vi "Curtin1.vi"() -> ()   [LabVIEW 2022 SP3]
uses:
  ViolinSubs/Curtin1_Label.ctl
  ViolinSubs/GraphType.ctl
  <vilib>/Utility/miscctls.llb/LVPoint32TypeDef.ctl
  ViolinSubs/Mic/Mic_Global.vi
  ViolinSubs/Perspective/subs/Perspective_Globals.vi
  <vilib>/Platform/browser.llb/Open URL in Default Browser (string).vi
panel:
  in  "microphone":bool
  in  "Device":u16(ring) items=["BuerginBase Microphone", "MacBook Pro Microphone", "Reincubate", "Microsoft Teams Audio", "Jump Desktop Microphone", "Jump Desktop Audio", "ZoomAudioDevice"]
  out "comma?":bool
  out "startX":i32
  out "Ctrl":bool
  out "beta":string
  in  "Settings":u16(ring) items=["Settings...", "Preferences", "Templates", "Calibrations", "Live View", "Motor Cntrl"]
  in  "ScratchPads":u16(ring) items=["Scratch...", "Admittance Scratchpad", "Radiation ScratchPad", "ScratchPad", "TapTones ScratchPad"]
  in  "New Test":u16(ring) items=["New Test...", "Admittance H", "JC H 12 radiation", "JC H 7 radiation", "JC HV 24 radiation"]
  in  "Help":bool
  in  "About":bool
  in  "Start":bool
  in  "email":bool
  in  "Interpret":bool
  in  "Force YRescale":bool
  out "Complex Out":cluster{dbl, "df":dbl, cdb[]}[](array[cluster])
  out "# selected":i32
  in  "Fun":bool
  out "Version":string
  in  "Preferences":bool
  in  "Set Colors":bool
  in  "Colors":u16(ring) items=["Name Current...", "Last Saved", "24 Colors"]
  in  "Share":bool
  in  "Undo":bool
  in  "Clear All":bool
  in  "select all":bool
  in  "deselect":bool
  in  "Clear":bool
  in  "Lists":bool
  in  "Browse":bool
  in  "Search":bool
  in  "Redo":bool
  in  "Files":T1[](array[typedef])
  in  "zoom":bool
  in  "Mouse Down?":bool
  in  "Views":T3={"View Type"=0, "Smoothing"=0, "Bands"=0, "Edit"=FALSE, "rescale Y"=FALSE, "rescale X"=FALSE, "X_Low"=0.0, "X_High"=0.0, "dB Range"=40.0, "Excel"=FALSE, "Y Scaling"=TRUE, "X Scaling"=TRUE, "Plot"=0} {"Plot" items=["FRF", "rad phase unwrapped", "deg phase unwrapped", "rad phase wrapped", "deg phase wrapped", "White Plots", "MJ Map", "Real and Imaginary"]; "Bands" items=["No Bands", "JC violin 200-7000 Flat (200-7000)", "JC violin (200-780-1740-2930-7000)", "JC violin (200-780-7000)"]; "Smoothing" items=["No smoothing"=0, "1/4 semitone"=25, "1/2 semitone"=50, "1 semitone"=100, "2 semitones"=200, "3 semitones"=300, "4 semitones"=400, "Octave"=1200, "Woodhouse"=19]; "View Type" items=["As measured"=0, "Normalize"=1, "Cplx Average"=3, "Real Average"=4, "Standard Deviation"=5]}
  out "Position":string
  in  "Color Table":T4(ring)=enum."Greyscale"
  out "MJPlot":dbl[][](graph)
  out "Coords":T5
  out "White Plots":picture
  out "FRF":cluster{"x0":dbl, "df":dbl, dbl[]}[](graph)
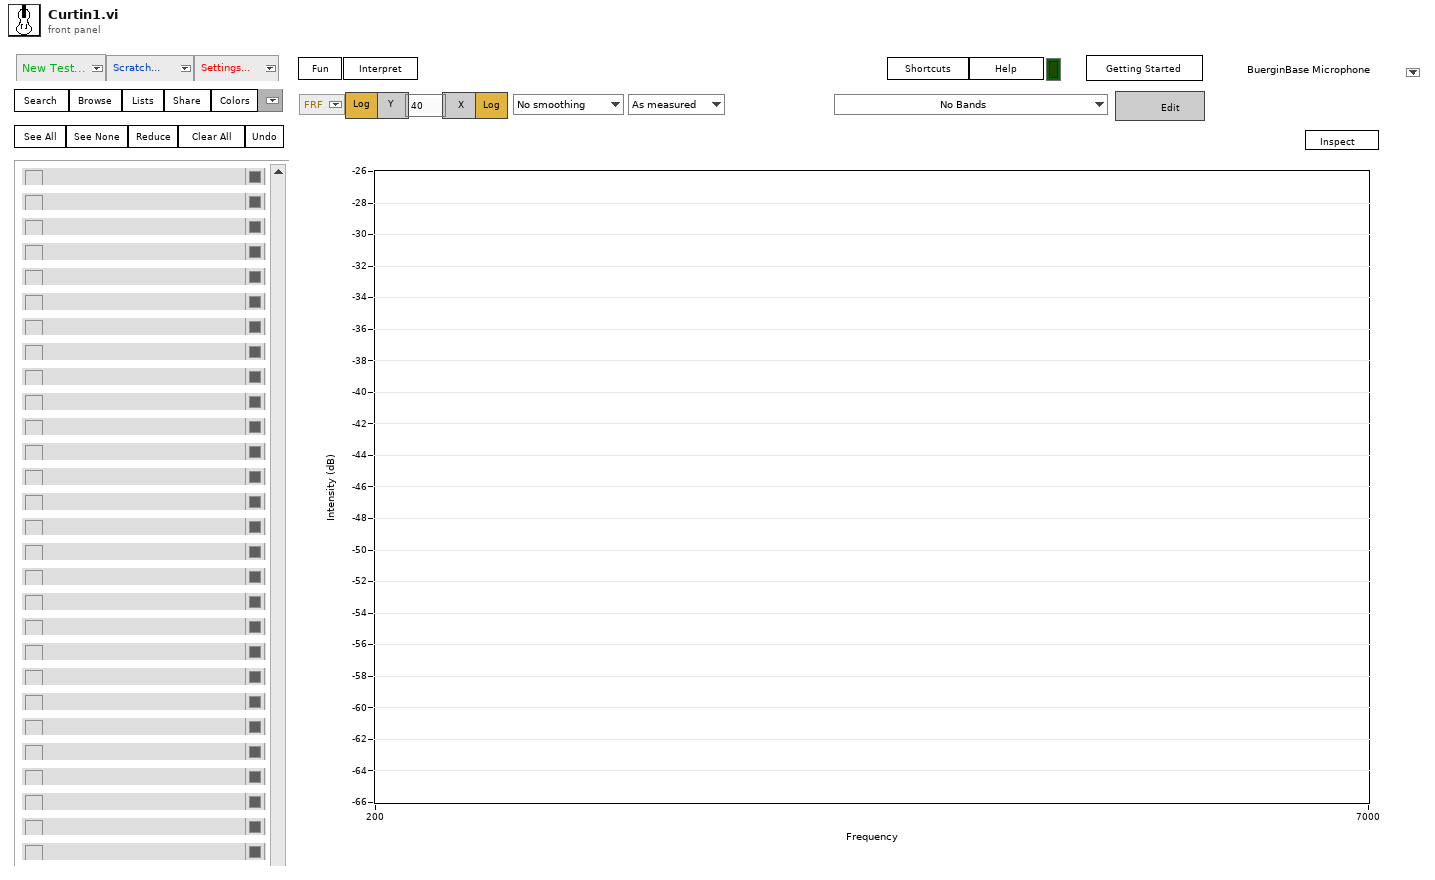
[diagram p1: front panel]
types:
  T1 = typedef "Curtin1_Label.ctl" = cluster{"Show?":bool, "Name":string, "Color":u32, "Path":path, "Show Notes":bool}
  T2 = typedef "GraphType.ctl" = u16
  T3 = cluster{"View Type":u16, "Smoothing":u16, "Bands":u16, "Edit":bool, "rescale Y":bool, "rescale X":bool, "X_Low":dbl, "X_High":dbl, "dB Range":dbl, "Excel":bool, "Y Scaling":bool, "X Scaling":bool, "Plot":T2}
  T4 = enum16{"Apricot", "Carnation", "Ether", "Greyscale", "Greyscale-banded", "Hot Metal", "Lava Waves", "Mac", "Morning Glory", "Rainbow", "Rainbow-banded", "Rainbow-inverted", "Rainbow-striped", "Saturn", "Seismic", "Space"}
  T5 = typedef "LVPoint32TypeDef.ctl" = cluster{"Horizontal":i32, "Vertical":i32}
  T6 = enum32{"SPL", "Voltage", "Accelerometer", "Vibrometer", "home", "Units"}
  T7 = enum16{"big-endian, network order", "native, host order", "little-endian"}
  T8 = enum16{"Grab Lines", "Grab Bands", "Grab Centroids"}
  T9 = cluster{"Alerts":bool, "Log X Axis":bool, "dB scale":bool, "Averaging":bool, "Fade":dbl, "Centroids?":bool}
  T10 = typedef "LVBoundsTypeDef.ctl" = cluster{"Width":u32, "Height":u32}
  T11 = typedef "LVPositionTypeDef.ctl" = cluster{"Left":i32, "Top":i32}
  T12 = typedef "PreferencesControl.ctl" = cluster{"Name of test":string, "Date":timestamp, "Location":string, "Template":string, "Soundcard":string, "resolution":u16, "Sampling rate":u16, "Ch1 Gain ":dbl, "Ch2 Gain":dbl, "Sample time (s)":dbl, "Pre-trigger (s)":dbl, "Hammer Threshold":dbl, "Positions":i16, "Taps/Position":i16, "Set Names":string, "Freq resolution":dbl, "Hammer cutoff":dbl, "Mic cutoff":dbl, "Double bounce ":dbl, "Hammer Cal":dbl, "dB Offset":dbl, "Accel Cal":dbl, "Vibrometer Cal":dbl, "Mic Cal":dbl, "Output":u16, "Voltage Cal":dbl, "Vibrometer Port":refnum<visa-resource-name>, "Range":u16, "High Pass":u16, "Bandwidth":u16, "X Range":cluster{"Minimum":dbl, "Maximum":dbl, "Increment":dbl, "Minor Increment":dbl, "Start":dbl}[], "Y Range":cluster{"Minimum":dbl, "Maximum":dbl, "Increment":dbl, "Minor Increment":dbl, "Start":dbl}[], "dB Spread":dbl, "Trigger":u16, "Ch_1":u8, "Ch_2":u8, "flip?":bool, "60Hz":bool, "Time offset":dbl, "Piezo Cal":dbl, "Default Notes":string}
  T13 = typedef "eventvkey.ctl" = enum16{"ASCII", "Enter", "Return", "Shift", "Ctrl", "Alt", "Cmd", "Opt", "Caps", "NumLock", "Clear", "Break", "Up", "Down", "Left", "Right", "Insert", "Delete", "Home", "End", "PageUp", "PageDown", "Escape", "Help", "Pause", "ScrollLock", "F1", "F2", "F3", "F4", "F5", "F6", "F7", "F8", "F9", "F10", "F11", "F12", "F13", "F14", "F15", "F16", "F17", "F18", "F19", "F20", "F21", "F22", "F23", "F24", "Play", "VolumeUp", "VolumeDown", "Mute", "Two Byte Char"}
  T14 = typedef "LVMouseTypeDef.ctl" = cluster{"Mouse Position":cluster{"X":i32, "Y":i32}, "Mouse Modifiers":cluster{"Button Down":bool, "Shift Mod":bool, "Menu Mod":bool, "Option Mod":bool}}
  T15 = enum32{"Invalid", "Standard", "Closed", "Hidden", "Minimized", "Maximized"}
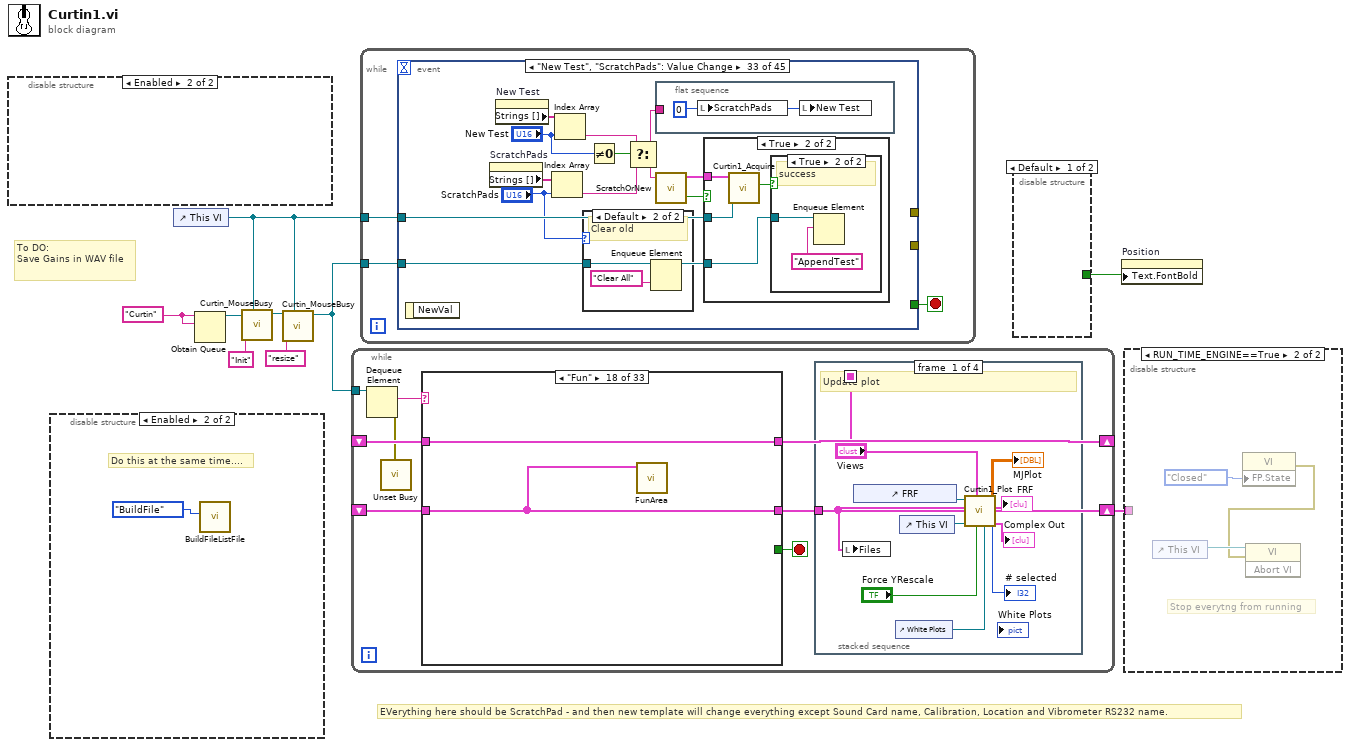
[diagram p0: block diagram]
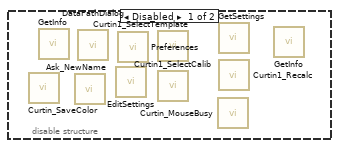
[diagram p2: hidden frame]
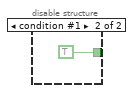
[diagram p4: hidden frame]
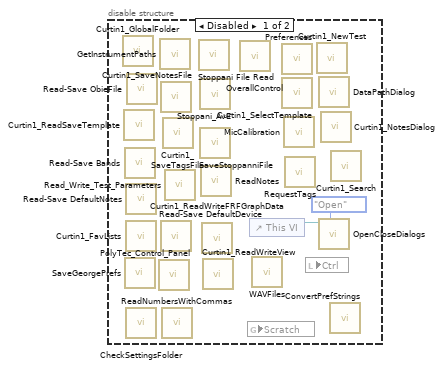
[diagram p5: hidden frame]
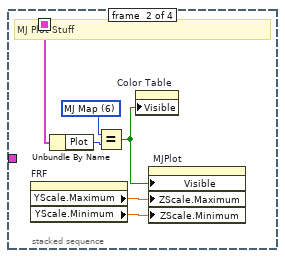
[diagram p6: hidden frame]
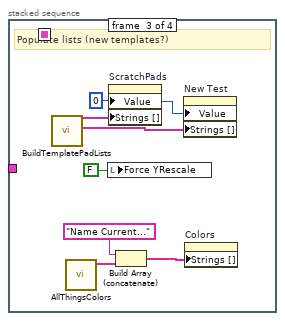
[diagram p7: hidden frame]
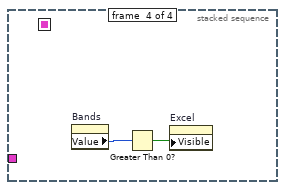
[diagram p8: hidden frame]
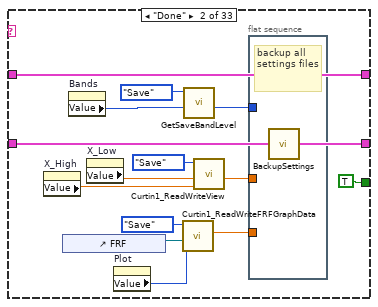
[diagram p10: hidden frame]
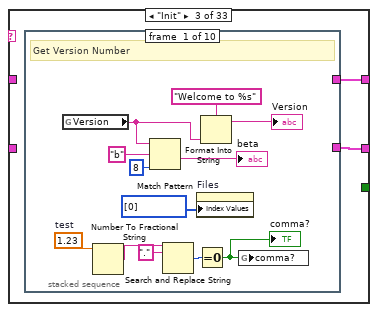
[diagram p11: hidden frame]
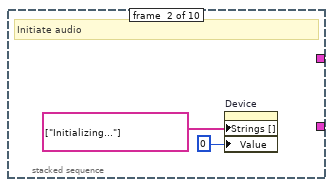
[diagram p12: hidden frame]
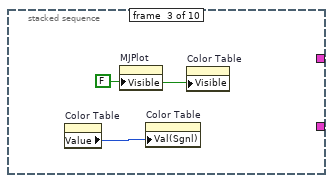
[diagram p13: hidden frame]
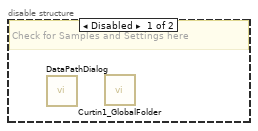
[diagram p15: hidden frame]
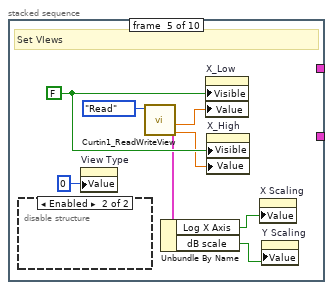
[diagram p16: hidden frame]
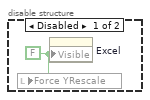
[diagram p17: hidden frame]
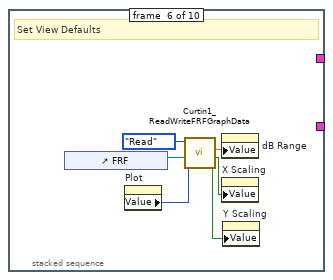
[diagram p18: hidden frame]
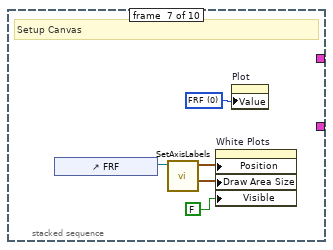
[diagram p19: hidden frame]
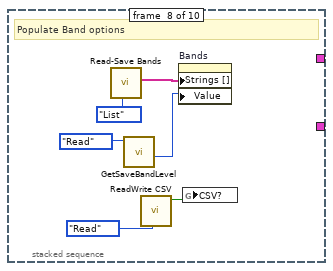
[diagram p20: hidden frame]
diagram:
  w7 = "Curtin" ("name (unnamed)")
  # "To DO:\nSave Gains in WAV file"
  # "EVerything here should be ScratchPad - and then new template will change everything except Sound Card name, Calibration, Location and Vibrometer RS232 name."
  n1 = disable-structure shown="Enabled" {
    frame Disabled {
      n2 = call "Curtin_SaveColor.vi"() -> ()  [unwired: 10 in, 2 out]
      n3 = call "GetInfo.vi"() -> ()  [unwired: 11 in, 1 out]
      n4 = call "Ask_NewName.vi"() -> ()  [unwired: 10 in, 2 out]
      n5 = call "DataPathDialog.vi"() -> ()  [unwired: 10 in, 2 out]
      n6 = call "EditSettings.vi"() -> ()  [unwired: 10 in, 2 out]
      n7 = call "Preferences.vi"() -> ()  [unwired: 9 in, 3 out]
      n8 = call "Curtin1_SelectTemplate.vi"() -> ()  [unwired: 10 in, 2 out]
      n9 = call "Curtin1_SelectCalib.vi"() -> ()  [unwired: 11 in, 1 out]
      n10 = call "Curtin_MouseBusy.vi"() -> ()  [unwired: 11 in, 1 out]
      n11 = call "GetSettings.vi"() -> ()  [unwired: 10 in, 2 out]
      n12 = call "Curtin1_Recalc.vi"() -> ()  [unwired: 12 in]
      n13 = call "GetInfo.vi"() -> ()  [unwired: 11 in, 1 out]
    }
    frame Enabled {
    }
  }
  n14 = disable-structure shown="Enabled" {
    frame Disabled {
      n15 = call "Curtin1_GlobalFolder.vi"() -> ()  [unwired: 1 in, 2 out]
      n16 = call "Curtin1_ReadSaveTemplate.vi"() -> ()  [unwired: 8 in, 4 out]
      n17 = call "Read-Save Bands.vi"() -> ()  [unwired: 8 in, 4 out]
      n18 = call "SaveGeorgePrefs.vi"() -> ()  [unwired: 10 in, 2 out]
      n19 = call "Read-Save DefaultNotes.vi"() -> ()  [unwired: 10 in, 2 out]
      n20 = call "Curtin1_FavLists.vi"() -> ()  [unwired: 8 in, 4 out]
      n21 = call "CheckSettingsFolder.vi"() -> ()  [unwired: 12 in]
      n22 = call "Read-Save ObieFile.vi"() -> ()  [unwired: 9 in, 3 out]
      n23 = call "PolyTec_Control_Panel.vi"() -> ()  [unwired: 9 in, 3 out]
      n24 = call "GetInstrumentPaths.vi"() -> ()  [unwired: 7 in, 5 out]
      n25 = call "Curtin1_SaveNotesFile.vi"() -> ()  [unwired: 12 in]
      n26 = call "Read-Save DefaultDevice.vi"() -> ()  [unwired: 10 in, 2 out]
      n27 = call "ReadNumbersWithCommas.vi"() -> ()  [unwired: 8 in, 4 out]
      n28 = call "Curtin1_SaveTagsFile.vi"() -> ()  [unwired: 12 in]
      n29 = call "Read_Write_Test_Parameters.vi"() -> ()  [unwired: 10 in, 2 out]
      n30 = call "Stoppani File Read.vi"() -> ()  [unwired: 3 in, 4 out]
      n31 = call "Stoppani_AvE.vi"() -> ()  [unwired: 8 in, 4 out]
      n32 = call "SaveStoppanniFile.vi"() -> ()  [unwired: 11 in, 1 out]
      n33 = call "ReadNotes.vi"() -> ()  [unwired: 10 in, 2 out]
      n34 = call "Curtin1_ReadWriteFRFGraphData.vi"() -> ()  [unwired: 9 in, 3 out]
      n35 = call "Curtin1_ReadWriteView.vi"() -> ()  [unwired: 9 in, 3 out]
      n36 = call "OverallControl.vi"() -> ()  [unwired: 10 in, 2 out]
      n37 = global read "Mic_Global.vi" "Scratch"() -> ()  [unwired: 1 in]
      n38 = control-ref of="This VI"() -> (w10:refnum<vi>)
      n39 = call "WAVFiles.vi"() -> ()  [unwired: 8 in, 4 out]
      n40 = call "Preferences.vi"() -> ()  [unwired: 9 in, 3 out]
      n41 = call "Curtin1_SelectTemplate.vi"() -> ()  [unwired: 10 in, 2 out]
      n42 = call "MicCalibration.vi"() -> ()  [unwired: 11 in, 1 out]
      n43 = call "RequestTags.vi"() -> ()  [unwired: 11 in, 1 out]
      n44 = local read "Ctrl"() -> ()  [unwired: 1 in]
      n45 = call "Curtin1_NewTest.vi"() -> ()  [unwired: 10 in, 2 out]
      n46 = call "DataPathDialog.vi"() -> ()  [unwired: 10 in, 2 out]
      n47 = call "OpenCloseDialogs.vi"("Task"=enum16{"Open", "Close"}."Open", "VI in"=w10) -> ()  [unwired: 8 in, 2 out]
      n48 = call "Curtin1_NotesDialog.vi"() -> ()  [unwired: 9 in, 3 out]
      n49 = call "ConvertPrefStrings.vi"() -> ()  [unwired: 10 in, 2 out]
      n50 = call "Curtin1_Search.vi"() -> ()  [unwired: 10 in, 2 out]
    }
    frame Enabled {
      # "Do this at the same time...."
      n51 = call "BuildFileListFile.vi"("Task"=enum16{"BuildFile", "ReadFile"}."BuildFile") -> ()  [unwired: 9 in, 2 out]
    }
  }
  n52 = control-ref of="This VI"() -> (w1:refnum<vi>)
  n53 = Obtain Queue(name (unnamed)=w7, element data type=w7) -> (queue out=w6:refnum<queue>)  [unwired: 3 in, 2 out]
  n54 = call "Curtin_MouseBusy.vi"("VI in"=w1, "element"="Init", "queue in"=w6) -> ("queue out"=w3:refnum<queue>)  [unwired: 8 in]
  n55 = call "Curtin_MouseBusy.vi"("VI in"=w1, "element"="resize", "queue in"=w3) -> ("queue out"=w4:refnum<queue>)  [unwired: 8 in]
  n56 = while {
    tunnel: w4 -> [w19]
    shift-right: [w16] -> w8
    shift-left: _ -> [w17]
    shift-right: [w14] -> _
    shift-left: _ -> [w15]
    stop <- w18 stop-if-true
    n57 = Dequeue Element(queue=w19) -> (element=w20:string, error out=w13:errorcluster)  [unwired: 2 in, 2 out]
    n58 = call <vilib>:"Unset Busy.vi"("error in (no error)"=w13) -> ()  [unwired: 10 in, 1 out]
    n59 = case shown="\"Fun\"" w20 {
      selector: w20 -> [_ _ _ _ _ _ _ _ _ _ _ _ _ _ _ _ _ _ _ _ _ _ _ _ _ _ _ _ _ _ w297 _ _]
      tunnel: [_ TRUE ("Discard?") _ _ _ _ _ _ _ _ _ _ _ _ _ _ _ _ _ _ _ _ _ _ _ _ _ _ _ _ _ _ _] -> w18
      tunnel: w17 -> [w47 w60 _ _ w124 w133 w149 w154 w156 w158 w160 w173 w180 w185 w196 w205 w218 w222 w224 w226 w230 w235 w238 w241 w254 w266 w272 w277 w282 w287 w298 w305 w328]
      tunnel: [w47 w60 w62 w112 w124 w135 w149 w154 w156 w158 w164 w172 w181 w187 w191 w205 w217 w222 w224 w226 w228 w234 w237 w241 w253 w265 w271 w279 T1[] [] ("Files") w289 w298 w305 w328] -> w16
      tunnel: [w46 w59 w63 w113 w127 w137 w150 w155 w157 w159 w162 w174 w182 w188 w197 w206 w220 w223 w225 w227 w231 w236 w239 w242 w255 w264 w270 w276 w283 w290 w299 w309 w329] -> w14
      tunnel: w15 -> [w46 w59 _ w114 w127 w137 w150 w155 w157 w159 w163 w175 w183 w189 w198 w206 w221 w223 w225 w227 w232 w236 w239 w242 w256 w264 w270 w278 w285 w288 w299 w309 w329]
      frame Default {
      }
      frame "Done" {
        n60 = property on="X_High" class="DigNum (strict)"() -> ("Value"=w54:dbl)  [unwired: 2 in, 2 out]
        n61 = control-ref of="FRF"() -> (w57:refnum<vi>)
        n62 = property on="Bands" class="Ring (strict)"() -> ("Value"=w52:u16)  [unwired: 2 in, 2 out]
        n63 = property on="X_Low" class="DigNum (strict)"() -> ("Value"=w55:dbl)  [unwired: 2 in, 2 out]
        n64 = property on="Plot" class="Ring (strict)"() -> ("Value"=w48:T2)  [unwired: 2 in, 2 out]
        n65 = call "Curtin1_ReadWriteFRFGraphData.vi"("Type"=w48, "FRF"=w57, "Task"=enum16{"Read", "Save"}."Save") -> ("dB"=w49:dbl)  [unwired: 6 in, 2 out]
        n66 = call "GetSaveBandLevel.vi"("Value in"=w52, "Task"=enum16{"Read", "Save"}."Save") -> ("Value out"=w51:u16)  [unwired: 9 in]
        n67 = call "Curtin1_ReadWriteView.vi"("X_High"=w54, "X_Low"=w55, "Task"=enum16{"Read", "Save"}."Save") -> ("X_Low out"=w50:dbl)  [unwired: 6 in, 2 out]
        n68 = flat-sequence {
          tunnel: w51 -> [_]
          tunnel: w50 -> [_]
          tunnel: w49 -> [_]
          frame #0 {
            # "backup all settings files"
            n69 = call "BackupSettings.vi"() -> ()  [unwired: 12 in]
          }
        }
      }
      frame "Init" {
        n70 = stacked-sequence {
          tunnel: [_ _ _ _ _ _ _ _ _ cluster{"files":T1[]}[] [] ("Array in")] -> w63
          tunnel: [_ _ _ _ _ _ _ _ _ T1[] [] ("Files")] -> w62
          frame #0 {
            w65 = 1.23  # test
            # "Get Version Number"
            n71 = global read "Mic_Global.vi" "Version"() -> (w69:string)
            n72 = Number To Fractional String(number=w65) -> (F-format string=w64:string)  [unwired: 3 in]
            n73 = Match Pattern(string=w69, regular expression="b", offset (0)=8) -> (after substring=→"beta":string)  [unwired: 3 out]
            n74 = Search and Replace String(input string=w64, search string=".") -> (number of replacements=w68:i32)  [unwired: 6 in, 3 out]
            n75 = property on="Files" class="Arr"("Index Values"=u32[] [0]) -> ()  [unwired: 2 in, 2 out]
            n76 = Equal To 0?(x=w68) -> (x = 0?=w66:bool)
            "comma?" <- w66
            n77 = Format Into String(format string="Welcome to %s", w69) -> (resulting string=→"Version":string)  [unwired: 2 in, 1 out]
            n78 = global write "Mic_Global.vi" "comma?"(w66) -> ()
          }
          frame #1 {
            # "Initiate audio"
            n79 = property on="Device" class="Ring (strict)"("Strings []"=string[] ["Initializing..."] ("Strings [4]"), "Value"=0) -> ()  [unwired: 2 in, 2 out]
          }
          frame #2 {
            w79 = FALSE ("Visible")
            n80 = property on="Color Table" class="Enum (strict)"() -> ("Value"=w78:T4)  [unwired: 2 in, 2 out]
            n81 = property on="MJPlot" class="IntGraph (strict)"("Visible"=w79) -> ()  [unwired: 2 in, 2 out]
            n82 = property on="Color Table" class="Enum (strict)"("Val(Sgnl)"=w78) -> ()  [unwired: 2 in, 2 out]
            n83 = property on="Color Table" class="Enum (strict)"("Visible"=w79) -> ()  [unwired: 2 in, 2 out]
          }
          frame #3 {
            # "Check Data Folder"
            n84 = disable-structure shown="Enabled" {
              frame Disabled {
                # "Check for Samples and Settings here"
                n85 = call "DataPathDialog.vi"() -> ()  [unwired: 10 in, 2 out]
                n86 = call "Curtin1_GlobalFolder.vi"() -> ()  [unwired: 1 in, 2 out]
              }
              frame Enabled {
              }
            }
          }
          frame #4 {
            w87 = FALSE ("Visible")
            # "Set VIews"
            n87 = disable-structure shown="Enabled" {
              frame Disabled {
                w88 = FALSE ("Visible")
                n88 = local write "Force YRescale"(w88) -> ()
                n89 = property on="Excel" class="Bool"("Visible"=w88) -> ()  [unwired: 2 in, 2 out]
              }
              frame Enabled {
              }
            }
            n90 = property on="View Type" class="Ring (strict)"("Value"=u16 0) -> ()  [unwired: 2 in, 2 out]
            n91 = call "Curtin1_ReadWriteView.vi"("Task"=enum16{"Read", "Save"}."Read") -> ("X_High out"=w84:dbl, "X_Low out"=w85:dbl, "View"=w80:T9)  [unwired: 8 in]
            n92 = Unbundle By Name(w80) -> ("Log X Axis"=w81:bool, "dB scale"=w82:bool)
            n93 = property on="X_Low" class="DigNum (strict)"("Visible"=w87, "Value"=w85) -> ()  [unwired: 2 in, 2 out]
            n94 = property on="X_High" class="DigNum (strict)"("Visible"=w87, "Value"=w84) -> ()  [unwired: 2 in, 2 out]
            n95 = property on="X Scaling" class="Bool (strict)"("Value"=w81) -> ()  [unwired: 2 in, 2 out]
            n96 = property on="Y Scaling" class="Bool (strict)"("Value"=w82) -> ()  [unwired: 2 in, 2 out]
          }
          frame #5 {
            # "Set View Defaults"
            n97 = control-ref of="FRF"() -> (w94:refnum<vi>)
            n98 = property on="Plot" class="Ring (strict)"() -> ("Value"=w91:T2)  [unwired: 2 in, 2 out]
            n99 = call "Curtin1_ReadWriteFRFGraphData.vi"("Type"=w91, "FRF"=w94, "Task"=enum16{"Read", "Save"}."Read") -> ("y log?"=w90:bool, "x log?"=w89:bool, "dB"=w92:dbl)  [unwired: 6 in]
            n100 = property on="dB Range" class="DigNum (strict)"("Value"=w92) -> ()  [unwired: 2 in, 2 out]
            n101 = property on="X Scaling" class="Bool (strict)"("Value"=w89) -> ()  [unwired: 2 in, 2 out]
            n102 = property on="Y Scaling" class="Bool (strict)"("Value"=w90) -> ()  [unwired: 2 in, 2 out]
          }
          frame #6 {
            w95 = T2 0 items=["FRF", "rad phase unwrapped", "deg phase unwrapped", "rad phase wrapped", "deg phase wrapped", "White Plots"] ("Value")
            # "Setup Canvas"
            n103 = control-ref of="FRF"() -> (w99:refnum<vi>)
            n104 = call "SetAxisLabels.vi"("WaveformGraph in"=w99) -> ("Bounds"=w97:T10, "Position"=w98:T11)  [unwired: 8 in, 1 out]
            n105 = property on="White Plots" class="Pict"("Position"=w98, "Draw Area Size"=w97, "Visible"=FALSE) -> ()  [unwired: 2 in, 2 out]
            n106 = property on="Plot" class="Ring (strict)"("Value"=w95) -> ()  [unwired: 2 in, 2 out]
          }
          frame #7 {
            # "Populate Band options"
            n107 = call "Read-Save Bands.vi"("Task"=enum16{"Save", "Read", "List"}."List") -> ("Long names"=w105:string[])  [unwired: 7 in, 3 out]
            n108 = call "GetSaveBandLevel.vi"("Task"=enum16{"Read", "Save"}."Read") -> ("Value out"=w102:u16)  [unwired: 10 in]
            n109 = call "ReadWrite CSV.vi"("Task"=enum16{"Save", "Read"}."Read") -> ("csv Out"=w100:bool)  [unwired: 10 in]
            n110 = property on="Bands" class="Ring (strict)"("Strings []"=w105, "Value"=w102) -> ()  [unwired: 2 in, 2 out]
            n111 = global write "Mic_Global.vi" "CSV?"(w100) -> ()
          }
          frame #8 {
            # "Always start everyone with ScratchPad \n\nRead the latest calibration but do not \ndo anything with it (no error code/saving)"
            # "Upload  ScratchPad template"
            n112 = call "UpdateScratchPad.vi"() -> ("Settings Out"=w107:T12)  [unwired: 10 in, 1 out]
            n113 = global write "Mic_Global.vi" "Settings"(w107) -> ()
            n114 = control-ref of="Device"() -> (w108:refnum<vi>)
            n115 = call "Curtin1_soundcards.vi"("hush?"=TRUE, "Settings In"=w107, "device:"=w108) -> ()  [unwired: 7 in, 2 out]
          }
          frame #9 {
            # "Initialize Undo and List"
          }
        }
      }
      frame "Update" {
        # "NOTE: info box is in this frame"
        n116 = call "Curtin1_NotesDialog.vi"("Files"="Files") -> ("Color"=w116:u32[], "removed?"=w115:bool, "Array"=w112:T1[])  [unwired: 8 in]
        n117 = call "Curtin1_Color.vi"("Color"=w116) -> ()  [unwired: 9 in, 2 out]
        n118 = case shown="True" w115 {
          tunnel: w114 -> [w118 w121]
          tunnel: [w118 w120] -> w113
          tunnel: w112 -> [_ w119]
          frame False {
          }
          frame True {
            # "removed a plot"
            n119 = call "Curtin_Undo.vi"("New Files"=w119, "Array in"=w121) -> ("Array out"=w120:cluster{"files":T1[]}[])  [unwired: 9 in]
          }
        }
        n120 = property on="Colors" class="Ring (strict)"("Value"=-1) -> ()  [unwired: 2 in, 2 out]
      }
      frame "Zoom" {
        n121 = for {
          tunnel: w124 -> [w130] mode=indexing
          tunnel: [w129] -> w123 mode=indexing if=w128
          n122 = Unbundle By Name(w130) -> ("Name"=w129:string, "Show?"=w128:bool)
        }
        n123 = property on="Plot" class="Ring (strict)"() -> ("Value"=w122:T2)  [unwired: 2 in, 2 out]
        n124 = property on="dB Range" class="DigNum (strict)"() -> ("Value"=w125:dbl)  [unwired: 2 in, 2 out]
        n125 = control-ref of="FRF"() -> (w126:refnum<vi>)
        n126 = call "GraphZoom.vi"("Plot"=w122, "Names"=w123, "dB Range"=w125, "Graph"=w126) -> ()  [unwired: 8 in]
      }
      frame "Preferences" {
        n127 = control-ref of="Files"() -> (w136:refnum<vi>)
        n128 = call "Preferences.vi"("FileList"=w136, "Files"=w133) -> ("Settings out"=w131:T12, "Success?"=w134:bool, "Fixed Files"=w132:T1[])  [unwired: 7 in]
        n129 = case shown="True" w134 {
          tunnel: w132 -> [_ w146]
          tunnel: [w138 w146] -> w135
          tunnel: w133 -> [w138 _]
          tunnel: w131 -> [_ w142]
          frame False {
          }
          frame True {
            n130 = global read "Mic_Global.vi" "View"() -> (w145:T9)
            n131 = call "UpdateScratchPad.vi"("Settings"=w142) -> ("Settings Out"=w139:T12)  [unwired: 9 in, 1 out]
            n132 = Unbundle By Name(w145) -> ("Log X Axis"=w144:bool, "dB scale"=w143:bool)
            n133 = control-ref of="Device"() -> (w141:refnum<vi>)
            n134 = call "Curtin1_soundcards.vi"("hush?"=TRUE, "Settings In"=w139, "device:"=w141) -> ()  [unwired: 7 in, 2 out]
            n135 = property on="X Scaling" class="Bool (strict)"("Value"=w144) -> ()  [unwired: 2 in, 2 out]
            n136 = property on="Y Scaling" class="Bool (strict)"("Value"=w143) -> ()  [unwired: 2 in, 2 out]
          }
        }
      }
      frame "Templates" {
        n137 = global read "Mic_Global.vi" "Scratch"() -> (w148:string)
        n138 = call "EditSettings.vi"("Template in"=w148) -> ("Settings out"=w147:T12)  [unwired: 9 in, 1 out]
        n139 = call "UpdateScratchPad.vi"("Settings"=w147) -> ()  [unwired: 9 in, 2 out]
      }
      frame "Calibrations" {
        # "Saves a new calib file\nand it is pushed in test"
        n140 = call "UpdateScratchPad.vi"() -> ("Settings Out"=w152:T12)  [unwired: 10 in, 1 out]
        n141 = call "MicCalibration.vi"("Type"=T6."home" ("Tyoe"), "Settings"=w152) -> ("Settings Out"=w151:T12)  [unwired: 9 in]
        n142 = global write "Mic_Global.vi" "Settings"(w151) -> ()
        n143 = call "UpdateScratchPad.vi"("Settings"=w151) -> ()  [unwired: 9 in, 2 out]
      }
      frame "LiveView" {
        n144 = call "LiveSignal.vi"() -> ()  [unwired: 12 in]
      }
      frame "MotorControl" {
        n145 = call "MotorControl.vi"() -> ()  [unwired: 12 in]
      }
      frame "Browse" {
        n146 = Array Size(array=w160) -> (size(s)=w161:i32)
        n147 = case shown="0" w161 {
          frame Default {
          }
          frame 0 {
            n148 = local write "Force YRescale"(TRUE ("Force YRescale")) -> ()
          }
        }
        n149 = call "Curtin_Undo.vi"("New Files"=w160, "Array in"=w163) -> ("Array out"=w162:cluster{"files":T1[]}[])  [unwired: 9 in]
        n150 = call "Curtin1_LoadFile.vi"("Files in"=w160) -> ("Files out"=w164:T1[])  [unwired: 10 in]
      }
      frame "Preload" {
        n151 = call "Curtin1_GlobalFolder.vi"() -> ("Samples"=w166:path)  [unwired: 1 in, 1 out]
        n152 = List Folder(path=w166, pattern="*.AvC") -> (path out=w169:path, filenames=w168:string[])  [unwired: 2 in, 2 out]
        n153 = call "Curtin_Undo.vi"("New Files"=w173, "Array in"=w175) -> ("Array out"=w174:cluster{"files":T1[]}[])  [unwired: 9 in]
        n154 = local write "Force YRescale"(TRUE ("Force YRescale")) -> ()
        n155 = for {
          tunnel: w169 -> [w178]
          tunnel: w168 -> [w177] mode=indexing
          tunnel: [w176] -> w167 mode=indexing
          n156 = Build Path(base path=w178, name or relative path=w177) -> (appended path=w176:path)
        }
        n157 = call "Curtin1_AddTest.vi"("Selected Paths"=w167) -> ("New Files"=w172:T1[])  [unwired: 10 in]
      }
      frame "Search" {
        n158 = Array Size(array=w180) -> (size(s)=w179:i32)
        n159 = case shown="0" w179 {
          frame Default {
          }
          frame 0 {
            n160 = local write "Force YRescale"(TRUE ("Force YRescale")) -> ()
          }
        }
        n161 = call "Curtin_Undo.vi"("New Files"=w180, "Array in"=w183) -> ("Array out"=w182:cluster{"files":T1[]}[])  [unwired: 9 in]
        n162 = call "Curtin1_Search.vi"("Old Files"=w180) -> ("New Files"=w181:T1[])  [unwired: 9 in, 1 out]
      }
      frame "Lists" {
        n163 = Array Size(array=w185) -> (size(s)=w186:i32)
        n164 = case shown="0" w186 {
          frame Default {
          }
          frame 0 {
            n165 = local write "Force YRescale"(TRUE ("Force YRescale")) -> ()
          }
        }
        n166 = call "Curtin_Undo.vi"("New Files"=w185, "Array in"=w189) -> ("Array out"=w188:cluster{"files":T1[]}[])  [unwired: 9 in]
        n167 = call "Curtin1_Lists.vi"("Old Files"=w185) -> ("New Files"=w187:T1[])  [unwired: 10 in]
      }
      frame "newColors" {
        n168 = property on="Colors" class="Ring (strict)"() -> ("Strings []"=w194:string[], "Value"=w195:u16)  [unwired: 2 in, 2 out]
        n169 = Index Array(array=w194, index=w195) -> (element=w193:string)
        n170 = call "AllThingsColors.vi"("Choice"=w193) -> ("Possible Colors"=w192:string[])  [unwired: 10 in]
        n171 = for {
          tunnel: w196 -> [w202] mode=indexing
          tunnel: [w201] -> w191 mode=indexing
          tunnel: w192 -> [_]
          i -> [w200]
          n172 = call "Curtin1_Color.vi"("Offset"=w200) -> ("New color"=w199:u32)  [unwired: 9 in, 1 out]
          n173 = Bundle By Name(cluster=w202, "Color"=w199) -> (w201:T1)
        }
        n174 = call "Curtin_Undo.vi"("New Files"=w196, "Array in"=w198) -> ("Array out"=w197:cluster{"files":T1[]}[])  [unwired: 9 in]
        n175 = local write "Files"(w191) -> ()
      }
      frame "saveColors" {
        n176 = call "Curtin_SaveColor.vi"() -> ("New Color"=w204:string, "Good?"=w203:bool)  [unwired: 10 in]
        n177 = case shown="True" w203 {
          tunnel: w205 -> [_ w209]
          tunnel: w204 -> [_ w208]
          tunnel: [_ w207] -> _
          frame False {
          }
          frame True {
            n178 = for {
              tunnel: w209 -> [w216] mode=indexing
              tunnel: [w215] -> w213 mode=indexing
              n179 = Unbundle By Name(w216) -> ("Color"=w215:u32)
            }
            n180 = call "Curtin1_GlobalFolder.vi"() -> ("LabVIEW Data Path"=w212:path)  [unwired: 1 in, 1 out]
            n181 = Build Path(base path=w212, name or relative path=w208) -> (appended path=w214:path)
            n182 = Write to Binary File(file (use dialog)=w214, data=w213, 5:FALSE ("prepend array or string size? (T)"), 9:T7."big-endian, network order" ("byte order (0:big-endian, network order)")) -> (error out=w207:errorcluster)  [unwired: 2 in, 2 out]
          }
        }
      }
      frame "setColors" {
        n183 = control-ref of="Files"() -> (w219:refnum<vi>)
        n184 = call "DefineColorPalette.vi"("Files in"=w218, "FileList"=w219) -> ("Files out"=w217:T1[])  [unwired: 9 in]
        n185 = call "Curtin_Undo.vi"("New Files"=w218, "Array in"=w221) -> ("Array out"=w220:cluster{"files":T1[]}[])  [unwired: 9 in]
      }
      frame "Fun" {
        n186 = call "FunArea.vi"("Old Files"=w222) -> ()  [unwired: 11 in]
      }
      frame "PlayIt" {
        n187 = call "PlayFile.vi"("Old Files"=w224) -> ()  [unwired: 11 in]
      }
      frame "Share" {
        n188 = call "Curtin1_Share.vi"("Files"=w226) -> ()  [unwired: 11 in]
      }
      frame "AppendTest" {
        n189 = global read "Mic_Global.vi" "Settings"() -> (w229:T12)
        n190 = call "Curtin1_DAQFiles.vi"("Settings"=w229, "Files in"=w230) -> ("Files out"=w228:T1[])  [unwired: 9 in]
        n191 = call "Curtin_Undo.vi"("New Files"=w230, "Array in"=w232) -> ("Array out"=w231:cluster{"files":T1[]}[])  [unwired: 9 in]
        n192 = flat-sequence {
          tunnel: w228 -> [_]
          frame #0 {
            n193 = call "BuildFileListFile.vi"("Task"=enum16{"BuildFile", "ReadFile"}."BuildFile") -> ()  [unwired: 9 in, 2 out]
          }
        }
      }
      frame "woodhouse" {
        n194 = call "Woodhouse.vi"("Files in"=w235) -> ("Files out"=w234:T1[])  [unwired: 10 in]
      }
      frame "SamZ" {
        n195 = call "SamZ_Format.vi"("Files in"=w238) -> ("Files out"=w237:T1[])  [unwired: 10 in]
      }
      frame "Folder" {
        n196 = for {
          tunnel: w241 -> [w247] mode=indexing
          tunnel: [w246] -> w240 mode=indexing if=w245
          n197 = Unbundle By Name(w247) -> ("Path"=w246:path, "Show?"=w245:bool)
        }
        n198 = for {
          tunnel: w240 -> [w244] mode=indexing
          n199 = Strip Path(path=w244) -> (stripped path=w243:path)  [unwired: 1 out]
          n200 = call "OpenFolder.vi"("LabVIEW Data Path"=w243) -> ()  [unwired: 11 in]
        }
      }
      frame "AppendAve" {
        n201 = local read "Complex Out"() -> (w252:cluster{dbl, "df":dbl, cdb[]}[])
        n202 = property on="View Type" class="Ring (strict)"() -> ("Value"=w250:u16)  [unwired: 2 in, 2 out]
        n203 = local read "# selected"() -> (w251:i32)
        n204 = call "SaveGroupAverages.vi"("nAverages"=w251, "Value"=w250, "Complex"=w252) -> ("New Path"=w248:path)  [unwired: 8 in]
        n205 = Not A Number/Path/Refnum?(number/path/refnum=w248) -> (NaN/Path/Refnum?=w249:bool)
        n206 = call "Curtin_Undo.vi"("New Files"=w254, "Array in"=w256) -> ("Array out"=w255:cluster{"files":T1[]}[])  [unwired: 9 in]
        n207 = case shown="False" w249 {
          tunnel: w254 -> [w261 w263]
          tunnel: [w260 w263] -> w253
          tunnel: w248 -> [w259 _]
          frame False {
            n208 = Build Array(w259) -> (w258:path[])
            n209 = call "Curtin1_AddTest.vi"("Old Files"=w261, "Selected Paths"=w258) -> ("New Files"=w260:T1[])  [unwired: 9 in]
            n210 = property on="View Type" class="Ring (strict)"("Val(Sgnl)"=0) -> ()  [unwired: 2 in, 2 out]
            n211 = call "BuildFileListFile.vi"("Task"=enum16{"BuildFile", "ReadFile"}."BuildFile") -> ()  [unwired: 9 in, 2 out]
          }
          frame True {
          }
        }
      }
      frame "Deselect" {
        n212 = for {
          tunnel: w266 -> [w269] mode=indexing
          tunnel: [w268] -> w265 mode=indexing
          n213 = Bundle By Name(cluster=w269, "Show?"=FALSE) -> (w268:T1)
        }
      }
      frame "SelectAll" {
        n214 = for {
          tunnel: w272 -> [w275] mode=indexing
          tunnel: [w274] -> w271 mode=indexing
          n215 = Bundle By Name(cluster=w275, "Show?"=TRUE) -> (w274:T1)
        }
      }
      frame "Clear" {
        n216 = call "Curtin_Undo.vi"("New Files"=w277, "Array in"=w278) -> ("Array out"=w276:cluster{"files":T1[]}[])  [unwired: 9 in]
        n217 = for {
          tunnel: w277 -> [w281] mode=indexing
          tunnel: [w281] -> w279 mode=indexing if=w280
          n218 = Unbundle By Name(w281) -> ("Show?"=w280:bool)
        }
      }
      frame "Clear All" {
        n219 = call "Curtin_Undo.vi"("New Files"=w282, "Array in"=w285) -> ("Array out"=w283:cluster{"files":T1[]}[])  [unwired: 9 in]
      }
      frame "Undo" {
        n220 = Array Size(array=w288) -> (size(s)=w286:i32)
        n221 = case shown="Default" w286 {
          tunnel: [w292 w296] -> w290
          tunnel: [w291 w293] -> w289
          tunnel: w288 -> [w292 w294]
          tunnel: w287 -> [w291 _]
          frame 0 {
          }
          frame Default {
            n222 = Delete From Array(array=w294) -> (deleted portion=w295:cluster{"files":T1[]}, array with subset deleted=w296:cluster{"files":T1[]}[])  [unwired: 2 in]
            n223 = Unbundle(w295) -> ("files"=w293:T1[])
          }
        }
      }
      frame "Left", "Right" {
        n224 = call "FadeLeftRight.vi"("Key"=w297) -> ()  [unwired: 11 in]
      }
      frame "BandEdit" {
        n225 = property on="Bands" class="Ring (strict)"() -> ("Strings []"=w307:string[], "Value"=w308:u16)  [unwired: 2 in, 2 out]
        n226 = for {
          tunnel: w305 -> [w314] mode=indexing
          tunnel: [w313] -> w304 mode=indexing if=w312
          n227 = Unbundle By Name(w314) -> ("Name"=w313:string, "Show?"=w312:bool)
        }
        n228 = Index Array(array=w307, index=w308) -> (element=w306:string)
        n229 = local read "FRF"() -> (w302:cluster{"x0":dbl, "df":dbl, dbl[]}[])
        n230 = Array Size(array=w304) -> (size(s)=w303:i32)
        n231 = call "ExtractBands.vi"("Task"=T8."Grab Lines", "lines"=w303, "plot in"=w302) -> ("plot out"=w301:cluster{dbl, "dt":dbl, "Y":dbl[]}[])  [unwired: 7 in, 1 out]
        n232 = call "BuildBandsList.vi"("Selected Band"=w306, "Average FRF"=w301) -> ("Name"=w311:string, "updated?"=w310:bool)  [unwired: 8 in]
        n233 = case shown="True" w310 {
          tunnel: w311 -> [_ w316]
          frame False {
          }
          frame True {
            n234 = call "Read-Save Bands.vi"("Task"=enum16{"Save", "Read", "List"}."List") -> ("Long names"=w317:string[])  [unwired: 7 in, 3 out]
            n235 = Search 1D Array(1D array=w317, element=w316) -> (index of element=w315:i32)  [unwired: 1 in]
            n236 = property on="Bands" class="Ring (strict)"("Strings []"=w317, "Value"=w315) -> ()  [unwired: 2 in, 2 out]
          }
        }
      }
      frame "resize" {
        n237 = property on="Show Notes" class="Bool"() -> ("Height"=w325:u32)  [unwired: 2 in, 2 out]
        n238 = property on="Pane 3" class="Pane"() -> ("Height"=w326:u32)  [unwired: 2 in, 2 out]
        n239 = control-ref of="FRF"() -> (w321:refnum<vi>)
        n240 = Add(x=u32 5, y=w325) -> (x+y=w324:u32)
        n241 = Divide(x=w326, y=w324) -> (x/y=w327:dbl)
        n242 = Round Toward -Infinity(1:w327) -> (0:w323:dbl)
        n243 = call "SetAxisLabels.vi"("WaveformGraph in"=w321) -> ("Bounds"=w319:T10, "Position"=w320:T11)  [unwired: 8 in, 1 out]
        n244 = property on="Files" class="Arr"("Number of Rows"=w323) -> ()  [unwired: 2 in, 2 out]
        n245 = property on="White Plots" class="Pict"("Position"=w320, "Draw Area Size"=w319) -> ()  [unwired: 2 in, 2 out]
      }
    }
    n246 = stacked-sequence {
      seq-local: ["Views" _ _ _] -> [_ w31 _ _]
      tunnel: w16 -> [w30 _ _ _]
      frame #0 {
        # "Update plot"
        n247 = local write "Files"(w30) -> ()
        n248 = control-ref of="FRF"() -> (w22:refnum<vi>)
        n249 = control-ref of="White Plots"() -> (w24:refnum<vi>)
        n250 = control-ref of="This VI"() -> (w28:refnum<vi>)
        n251 = call "Curtin1_Plot.vi"("Canvas 2"=w24, "Force YRescale"="Force YRescale", "Settings"="Views", "VI Refnum"=w28, "Files"=w30, "FRF"=w22) -> ("Complex Out"=→"Complex Out":cluster{dbl, "df":dbl, cdb[]}[], "size(s)"=→"# selected":i32, "Average FRF"=→"FRF":cluster{"x0":dbl, "df":dbl, dbl[]}[], "MJ Plot"=→"MJPlot":dbl[][])  [unwired: 2 in]
      }
      frame #1 {
        w35 = T2 6 items=["FRF", "rad phase unwrapped", "deg phase unwrapped", "rad phase wrapped", "deg phase wrapped", "White Plots", "MJ Map"] ("x")
        # "MJ Plot Stuff"
        n252 = property on="FRF" class="WFGraph (strict)"() -> ("YScale.Maximum"=w33:dbl, "YScale.Minimum"=w32:dbl)  [unwired: 2 in, 2 out]
        n253 = Unbundle By Name(w31) -> ("Plot"=w34:T2)
        n254 = Equal?(x=w35, y=w34) -> (x = y?=w36:bool)
        n255 = property on="Color Table" class="Enum (strict)"("Visible"=w36) -> ()  [unwired: 2 in, 2 out]
        n256 = property on="MJPlot" class="IntGraph (strict)"("Visible"=w36, "ZScale.Maximum"=w33, "ZScale.Minimum"=w32) -> ()  [unwired: 2 in, 2 out]
      }
      frame #2 {
        w37 = 0
        # "Populate lists (new templates?)"
        n257 = call "BuildTemplatePadLists.vi"() -> ("Templates"=w43:string[], "ScratchPads"=w38:string[])  [unwired: 8 in, 2 out]
        n258 = call "AllThingsColors.vi"() -> ("Possible Colors"=w41:string[])  [unwired: 11 in]
        n259 = local write "Force YRescale"(FALSE ("Force YRescale")) -> ()
        n260 = property on="ScratchPads" class="Ring (strict)"("Value"=w37, "Strings []"=w38) -> ()  [unwired: 2 in, 2 out]
        n261 = Build Array (concatenate)("Name Current...", w41) -> (w39:string[])
        n262 = property on="New Test" class="Ring (strict)"("Value"=w37, "Strings []"=w43) -> ()  [unwired: 2 in, 2 out]
        n263 = property on="Colors" class="Ring (strict)"("Strings []"=w39) -> ()  [unwired: 2 in, 2 out]
      }
      frame #3 {
        n264 = property on="Bands" class="Ring (strict)"() -> ("Value"=w45:u16)  [unwired: 2 in, 2 out]
        n265 = Greater Than 0?(x=w45) -> (x > 0?=w44:bool)
        n266 = property on="Excel" class="Bool"("Visible"=w44) -> ()  [unwired: 2 in, 2 out]
      }
    }
  }
  n267 = while {
    tunnel: w4 -> [w332]
    tunnel: w1 -> [w330]
    stop <- w331 stop-if-true
    n268 = event shown="[32] \"New Test\", \"ScratchPads\": Value Change" {
      selector: _ -> [_ _ _ _ _ _ _ _ _ _ _ _ _ _ _ _ _ _ _ _ _ _ _ _ _ _ _ _ _ _ _ _ _ _ _ _ _ _ _ _ _ _ _ _ _]
      dyn-events: _ -> [_ _ _ _ _ _ _ _ _ _ _ _ _ _ _ _ _ _ _ _ _ _ _ _ _ _ _ _ _ _ _ _ _ _ _ _ _ _ _ _ _ _ _ _ _]
      timeout: _ -> [_ _ _ _ _ _ _ _ _ _ _ _ _ _ _ _ _ _ _ _ _ _ _ _ _ _ _ _ _ _ _ _ _ _ _ _ _ _ _ _ _ _ _ _ _]
      tunnel: w332 -> [_ w333 w340 _ w351 w353 w356 w359 w363 w366 w369 w371 w375 w378 w381 w384 w387 w398 w413 _ w428 _ w446 _ w466 _ _ _ _ w498 _ _ w511 w535 _ w548 w553 w555 _ _ _ w565 w570 _ w577]
      tunnel: [_ w335 _ _ _ _ _ _ _ _ _ _ _ _ _ _ _ _ _ _ _ _ _ _ _ _ _ _ _ _ _ _ _ _ _ _ _ _ _ _ _ _ _ _ _] -> w331
      tunnel: w330 -> [_ w334 _ _ w350 w354 w355 w358 w361 w364 w367 w372 w374 w377 w379 w383 w385 w396 _ _ _ _ _ _ w465 _ _ _ _ _ _ _ w520 w534 _ w547 _ _ _ _ _ _ w571 _ _]
      tunnel: [_ _ _ _ _ _ _ _ _ _ _ _ _ _ _ _ _ _ _ _ _ _ _ _ _ _ _ _ _ _ _ _ _ _ _ _ _ _ _ _ _ _ _ w574 _] -> _
      tunnel: [_ _ _ _ _ _ _ _ _ _ _ _ _ _ _ _ _ _ _ w418 _ _ _ _ _ _ _ _ _ _ _ _ _ _ _ _ _ _ _ _ _ _ _ _ _] -> _
      event Timeout {
        n269 = event-data() -> ()  [unwired: 1 in, 3 out]
      }
      event Panel Close? {
        w335 = TRUE ("Discard?")
        n270 = event-data() -> ()  [unwired: 1 in, 4 out]
        n271 = call "Curtin_MouseBusy.vi"("VI in"=w334, "element"="Done", "queue in"=w333) -> ()  [unwired: 8 in, 1 out]
        n272 = event-data("Discard?"=w335) -> ()  [unwired: 1 in, 1 out]
      }
      event Key Down {
        n273 = event-data() -> ("VKey"=w341:T13, "PlatMods.Opt"=w339:bool, "PlatMods.Alt"=w338:bool)  [unwired: 1 in]
        n274 = Or(x=w339, y=w338) -> (x .or. y?=→"Ctrl":bool)
        n275 = case shown="\"Left\"" w341 {
          tunnel: w340 -> [_ w342 w344]
          frame Default {
          }
          frame "Left" {
            n276 = Enqueue Element(queue=w342, element="Left") -> ()  [unwired: 2 in, 3 out]
          }
          frame "Right" {
            n277 = Enqueue Element(queue=w344, element="Right") -> ()  [unwired: 2 in, 3 out]
          }
        }
      }
      event Key Up {
        n278 = event-data() -> ("PlatMods.Alt"=w348:bool, "PlatMods.Opt"=w347:bool)  [unwired: 1 in]
        n279 = Or(x=w348, y=w347) -> (x .or. y?=w346:bool)
        n280 = local write "Ctrl"(w346) -> ()
      }
      event Panel Resize {
        n281 = event-data() -> ()  [unwired: 1 in, 1 out]
        n282 = call "Curtin_MouseBusy.vi"("VI in"=w350, "element"="resize", "queue in"=w351) -> ()  [unwired: 8 in, 1 out]
      }
      event "Browse": Value Change {
        n283 = event-data() -> ()  [unwired: 1 in, 1 out]
        n284 = call "Curtin_MouseBusy.vi"("VI in"=w354, "element"="Browse", "queue in"=w353) -> ()  [unwired: 8 in, 1 out]
      }
      event "Search": Value Change {
        n285 = event-data() -> ()  [unwired: 1 in, 1 out]
        n286 = call "Curtin_MouseBusy.vi"("VI in"=w355, "element"="Search", "queue in"=w356) -> ()  [unwired: 8 in, 1 out]
      }
      event "deselect": Value Change {
        n287 = event-data() -> ()  [unwired: 1 in, 1 out]
        n288 = call "Curtin_MouseBusy.vi"("VI in"=w358, "element"="Deselect", "queue in"=w359) -> ()  [unwired: 8 in, 1 out]
      }
      event "select all": Value Change {
        n289 = event-data() -> ()  [unwired: 1 in, 1 out]
        n290 = call "Curtin_MouseBusy.vi"("VI in"=w361, "element"="SelectAll", "queue in"=w363) -> ()  [unwired: 8 in, 1 out]
      }
      event "Undo": Value Change {
        n291 = event-data() -> ()  [unwired: 1 in, 1 out]
        n292 = call "Curtin_MouseBusy.vi"("VI in"=w364, "element"="Undo", "queue in"=w366) -> ()  [unwired: 8 in, 1 out]
      }
      event "Redo": Value Change {
        n293 = event-data() -> ()  [unwired: 1 in, 1 out]
        n294 = call "Curtin_MouseBusy.vi"("VI in"=w367, "element"="Redo", "queue in"=w369) -> ()  [unwired: 8 in, 1 out]
      }
      event "Clear": Value Change {
        n295 = event-data() -> ()  [unwired: 1 in, 1 out]
        n296 = call "Curtin_MouseBusy.vi"("VI in"=w372, "element"="Clear", "queue in"=w371) -> ()  [unwired: 8 in, 1 out]
      }
      event "Files": Value Change {
        n297 = event-data() -> ()  [unwired: 1 in, 1 out]
        n298 = call "Curtin_MouseBusy.vi"("VI in"=w374, "element"="Update", "queue in"=w375) -> ()  [unwired: 8 in, 1 out]
      }
      event "Clear All": Value Change {
        n299 = event-data() -> ()  [unwired: 1 in, 3 out]
        n300 = call "Curtin_MouseBusy.vi"("VI in"=w377, "element"="Clear All", "queue in"=w378) -> ()  [unwired: 8 in, 1 out]
      }
      event "Lists": Value Change {
        n301 = event-data() -> ()  [unwired: 1 in, 1 out]
        n302 = call "Curtin_MouseBusy.vi"("VI in"=w379, "element"="Lists", "queue in"=w381) -> ()  [unwired: 8 in, 1 out]
      }
      event "Share": Value Change {
        n303 = event-data() -> ()  [unwired: 1 in, 1 out]
        n304 = call "Curtin_MouseBusy.vi"("VI in"=w383, "element"="Share", "queue in"=w384) -> ()  [unwired: 8 in, 1 out]
      }
      event "Colors": Value Change {
        n305 = event-data() -> ()  [unwired: 1 in, 2 out]
        n306 = case shown="0" "Colors" {
          tunnel: w387 -> [w390 w395]
          tunnel: w385 -> [w388 w391]
          frame 0 {
            n307 = call "Curtin_MouseBusy.vi"("VI in"=w388, "element"="saveColors", "queue in"=w390) -> ()  [unwired: 8 in, 1 out]
          }
          frame Default {
            n308 = call "Curtin_MouseBusy.vi"("VI in"=w391, "element"="newColors", "queue in"=w395) -> ("queue out"=w393:refnum<queue>)  [unwired: 8 in]
            n309 = call "Curtin_MouseBusy.vi"("VI in"=w391, "element"="Update", "queue in"=w393) -> ()  [unwired: 8 in, 1 out]
          }
        }
      }
      event "Set Colors": Value Change {
        n310 = event-data() -> ()  [unwired: 1 in, 1 out]
        n311 = call "Curtin_MouseBusy.vi"("VI in"=w396, "element"="setColors", "queue in"=w398) -> ()  [unwired: 8 in, 1 out]
        n312 = disable-structure shown="Disabled" {
          disable-tunnel: _ -> [w399 _]
          frame Disabled {
            n313 = Enqueue Element(queue=w399, element="Update") -> ()  [unwired: 2 in, 3 out]
          }
          frame Enabled {
          }
        }
      }
      event "Views": Value Change {
        n314 = event-data() -> ("NewVal"=w401:T3)  [unwired: 1 in]
        n315 = Unbundle By Name(w401) -> ("X Scaling"=w408:bool, "Y Scaling"=w407:bool, "View Type"=w412:u16, "Edit"=w403:bool)
        n316 = global read "Mic_Global.vi" "View"() -> (w409:T9)
        n317 = Bundle By Name(cluster=w409, "Log X Axis"=w408, "dB scale"=w407) -> (w406:T9)
        n318 = Select(t="BandEdit" ("element"), s=w403, f="Update" ("element")) -> (s? t:f=w402:string)
        n319 = Enqueue Element(queue=w413, element=w402) -> ()  [unwired: 2 in, 3 out]
        n320 = global write "Mic_Global.vi" "View"(w406) -> ()
        n321 = Equal?(x=u16 1 ("View Type"), y=w412) -> (x = y?=w410:bool)
        n322 = property on="X_Low" class="DigNum (strict)"("Visible"=w410) -> ()  [unwired: 2 in, 2 out]
        n323 = property on="X_High" class="DigNum (strict)"("Visible"=w410) -> ()  [unwired: 2 in, 2 out]
      }
      event "Views.dB Range": Value Change {
        n324 = event-data() -> ()  [unwired: 1 in, 1 out]
        n325 = control-ref of="FRF"() -> (w417:refnum<vi>)
        n326 = property class="WFGraph (strict)"(reference=w417) -> (reference out=w420:refnum<vi>, error out=w419:errorcluster, "YScale.Maximum"=w423:dbl)  [unwired: 1 in]
        n327 = property on="dB Range" class="DigNum (strict)"() -> ("Value"=w422:dbl)  [unwired: 2 in, 2 out]
        n328 = Subtract(x=w423, y=w422) -> (x-y=w421:dbl)
        n329 = property class="WFGraph (strict)"(reference=w420, error in=w419, "YScale.Minimum"=w421) -> (reference out=w416:refnum<vi>, error out=w418:errorcluster)
        n330 = property on="Plot" class="Ring (strict)"() -> ("Value"=w415:T2)  [unwired: 2 in, 2 out]
        n331 = call "Curtin1_ReadWriteFRFGraphData.vi"("Type"=w415, "FRF"=w416, "Task"=enum16{"Read", "Save"}."Save") -> ()  [unwired: 6 in, 3 out]
      }
      event "Views.View Type": Value Change {
        n332 = event-data() -> ("NewVal"=w425:u16)  [unwired: 1 in]
        n333 = disable-structure shown="Disabled" {
          disable-tunnel: w428 -> [w429 _]
          frame Disabled {
            n334 = Enqueue Element(queue=w429, element="Update") -> ()  [unwired: 2 in, 3 out]
          }
          frame Enabled {
          }
        }
        n335 = Equal?(x=u16 1 ("View Type"), y=w425) -> (x = y?=w427:bool)
        n336 = property on="X_Low" class="DigNum (strict)"("Visible"=w427) -> ()  [unwired: 2 in, 2 out]
        n337 = property on="X_High" class="DigNum (strict)"("Visible"=w427) -> ()  [unwired: 2 in, 2 out]
        n338 = local write "Force YRescale"(TRUE ("Force YRescale")) -> ()
      }
      event Value Change {
        n339 = event-data() -> ("NewVal"=w431:T2, "OldVal"=w432:T2)  [unwired: 1 in]
        n340 = stacked-sequence {
          tunnel: w432 -> [w433 _]
          tunnel: w431 -> [_ w437]
          frame #0 {
            n341 = control-ref of="FRF"() -> (w435:refnum<vi>)
            n342 = call "Curtin1_ReadWriteFRFGraphData.vi"("Type"=w433, "FRF"=w435, "Task"=enum16{"Read", "Save"}."Save") -> ()  [unwired: 6 in, 3 out]
          }
          frame #1 {
            w438 = T2 5 items=["FRF", "rad phase unwrapped", "deg phase unwrapped", "rad phase wrapped", "deg phase wrapped", "White Plots"] ("y")
            # "There is a bug in LV so runs twice\none for changing Views and again\nfor changing scaling value..."
            n343 = control-ref of="FRF"() -> (w441:refnum<vi>)
            n344 = Equal?(x=w437, y=w438) -> (x = y?=w439:bool)
            n345 = call "Curtin1_ReadWriteFRFGraphData.vi"("Type"=w437, "FRF"=w441, "Task"=enum16{"Read", "Save"}."Read") -> ("y log?"=w444:bool, "x log?"=w443:bool, "dB"=w442:dbl)  [unwired: 6 in]
            n346 = property on="White Plots" class="Pict"("Visible"=w439) -> ()  [unwired: 2 in, 2 out]
            n347 = property on="dB Range" class="DigNum (strict)"("Value"=w442) -> ()  [unwired: 2 in, 2 out]
            n348 = property on="X Scaling" class="Bool (strict)"("Value"=w443) -> ()  [unwired: 2 in, 2 out]
            n349 = local write "Force YRescale"(TRUE ("Force YRescale")) -> ()
            n350 = property on="Y Scaling" class="Bool (strict)"("Val(Sgnl)"=w444) -> ()  [unwired: 2 in, 2 out]
          }
        }
      }
      event "White Plots": Mouse Move {
        n351 = event-data() -> ()  [unwired: 1 in, 1 out]
        n352 = property on="White Plots" class="Pict"() -> ("Width"=w447:u32, "Mouse"=w449:T14)  [unwired: 2 in, 2 out]
        n353 = Unbundle By Name(w449) -> ("Mouse Position.X"=w445:i32, "Mouse Modifiers.Button Down"=w448:bool)
        n354 = case shown="True" w448 {
          tunnel: w445 -> [_ w460]
          tunnel: w447 -> [_ w459]
          tunnel: w446 -> [_ w457]
          tunnel: w445 -> [_ w456]
          frame False {
          }
          frame True {
            n355 = local read "startX"() -> (w455:i32)
            n356 = Divide(x=w460, y=w459) -> ()  [unwired: 1 out]
            n357 = Subtract(x=w456, y=w455) -> (x-y=w454:i32)
            n358 = Enqueue Element(queue=w457, element="Update") -> ()  [unwired: 2 in, 3 out]
            n359 = Bundle(w454, "y"=0) -> (w451:cluster{i32, "y":i32})  [unwired: 1 in]
            n360 = Add(x=cluster{"x":dbl, "y":dbl}[] [{"x"=-400.0, "y"=200.0}, {"x"=400.0, "y"=200.0}] ("vanishing points"), y=w451) -> (x+y=w450:cluster{dbl, "y":dbl}[])
            n361 = global write "Perspective_Globals.vi" "vanishing points"(w450) -> ()
          }
        }
      }
      event "White Plots": Mouse Down; "White Plots": Mouse Enter {
        n362 = event-data() -> ()  [unwired: 1 in, 4 out]
        n363 = property on="White Plots" class="Pict" props=["Width", "Mouse"]() -> ("Mouse"=w463:T14)  [unwired: 2 in, 3 out]
        n364 = Unbundle By Name(w463) -> ("Mouse Position.X"=→"startX":i32, "Mouse Modifiers.Button Down"=w462:bool)
        n365 = global write "Perspective_Globals.vi" "Outlines?"(w462) -> ()
      }
      event "White Plots": Mouse Leave; "White Plots": Mouse Up {
        n366 = event-data() -> ()  [unwired: 1 in, 1 out]
        n367 = call "Curtin_MouseBusy.vi"("VI in"=w465, "element"="Update", "queue in"=w466) -> ()  [unwired: 8 in, 1 out]
        n368 = global write "Perspective_Globals.vi" "Outlines?"(FALSE ("Outlines?")) -> ()
      }
      event "Color Table": Value Change {
        n369 = event-data() -> ()  [unwired: 1 in, 6 out]
        n370 = call "ColorTables.vi"("Color Table"="Color Table") -> ("Color Table Out"=w471:u32[])  [unwired: 2 in]
        n371 = property on="MJPlot" class="IntGraph (strict)"("Color Table"=w471, "ZScale.Low Color"=u32 16777215 ("Z Scale.Low Color"), "ZScale.Interpolate Color"=TRUE ("Z Scale.Interpolate Color"), "ZScale.High Color"=u32 0 ("Z Scale.High Color")) -> ()  [unwired: 2 in, 2 out]
      }
      event "FRF": Mouse Move {
        n372 = event-data() -> ("CtlRef"=w478:refnum<vi>, "Coords"=w477:T5)  [unwired: 1 in]
        n373 = local read "Coords"() -> (w473:T5)
        n374 = property on="Plot" class="Ring (strict)"() -> ("Value"=w474:T2)  [unwired: 2 in, 2 out]
        n375 = case shown="True" "Mouse Down?" {
          tunnel: w478 -> [_ w485]
          tunnel: w477 -> [_ w481]
          tunnel: ["" ("Position") w484] -> w476
          tunnel: w474 -> [_ w482]
          tunnel: w473 -> [_ w480]
          frame False {
          }
          frame True {
            n376 = local read "Ctrl"() -> (w483:bool)
            n377 = call "Cursor Values.vi"("Plot"=w482, "option?"=w483, "Start Coord"=w480, "Coords"=w481, "WaveformGraph in"=w485) -> ("Position"=w484:string)  [unwired: 6 in]
          }
        }
        "Position" <- w476
      }
      event "FRF": Mouse Enter {
        n378 = event-data() -> ()  [unwired: 1 in, 1 out]
        n379 = local write "Mouse Down?"(TRUE ("Mouse Down?")) -> ()
      }
      event "FRF": Mouse Leave {
        n380 = event-data() -> ()  [unwired: 1 in, 1 out]
        n381 = local write "Mouse Down?"(FALSE ("Mouse Down?")) -> ()
        n382 = local write "Coords"(T5 {"Horizontal"=0, "Vertical"=0} ("Coords")) -> ()
        n383 = property on="FRF" class="WFGraph (strict)"("Active Cursor"=u32 0, "Cursor.Visible"=FALSE) -> ()  [unwired: 2 in, 2 out]
        n384 = property on="FRF" class="WFGraph (strict)"("Active Cursor"=u32 1, "Cursor.Visible"=FALSE) -> ()  [unwired: 2 in, 2 out]
      }
      event "FRF": Mouse Up {
        n385 = event-data() -> ("PlatMods.Shift"=w499:bool)  [unwired: 1 in]
        n386 = local write "Coords"(T5 {"Horizontal"=0, "Vertical"=0} ("Coords")) -> ()
        n387 = case shown="True" w499 {
          tunnel: w498 -> [_ w500]
          frame False {
          }
          frame True {
            n388 = Enqueue Element(queue=w500, element="Zoom") -> ()  [unwired: 2 in, 3 out]
          }
        }
        n389 = property on="FRF" class="WFGraph (strict)"("Active Cursor"=u32 0, "Cursor.Visible"=FALSE) -> ()  [unwired: 2 in, 2 out]
        n390 = property on="FRF" class="WFGraph (strict)"("Active Cursor"=u32 1, "Cursor.Visible"=FALSE) -> ()  [unwired: 2 in, 2 out]
      }
      event "FRF": Mouse Down {
        n391 = event-data() -> ("PlatMods.Ctrl"=w504:bool, "Coords"=→"Coords":T5)  [unwired: 1 in]
        n392 = Not(x=w504) -> (.not. x?=w502:bool)
        n393 = disable-structure shown="Disabled" {
          disable-tunnel: w502 -> [w505 _]
          frame Disabled {
            n394 = property on="FRF" class="WFGraph (strict)"("Active Cursor"=u32 0, "Cursor.Visible"=w505) -> ()  [unwired: 2 in, 2 out]
            n395 = property on="FRF" class="WFGraph (strict)"("Active Cursor"=u32 1, "Cursor.Visible"=w505) -> ()  [unwired: 2 in, 2 out]
          }
          frame Enabled {
          }
        }
      }
      event "FRF": Scale Range Change {
        n396 = event-data() -> ("CtlRef"=w509:refnum<vi>)  [unwired: 1 in]
        n397 = property on="Plot" class="Ring (strict)"() -> ("Value"=w508:T2)  [unwired: 2 in, 2 out]
        n398 = call "Curtin1_ReadWriteFRFGraphData.vi"("Type"=w508, "FRF"=w509, "Task"=enum16{"Read", "Save"}."Save") -> ()  [unwired: 6 in, 3 out]
      }
      event "New Test", "ScratchPads": Value Change {
        n399 = event-data() -> ()  [unwired: 1 in, 1 out]
        n400 = property on="ScratchPads" class="Ring (strict)"() -> ("Strings []"=w519:string[])  [unwired: 2 in, 2 out]
        n401 = property on="New Test" class="Ring (strict)"() -> ("Strings []"=w518:string[])  [unwired: 2 in, 2 out]
        n402 = Index Array(array=w519, index="ScratchPads") -> (element=w515:string)
        n403 = Index Array(array=w518, index="New Test") -> (element=w516:string)
        n404 = case shown="Default" "ScratchPads" {
          tunnel: w511 -> [_ w524]
          frame 0 {
            # "New Test"
          }
          frame Default {
            # "Clear old"
            n405 = Enqueue Element(queue=w524, element="Clear All") -> ()  [unwired: 2 in, 3 out]
          }
        }
        n406 = Not Equal To 0?(x="New Test") -> (x != 0?=w517:bool)
        n407 = Select(t=w516, s=w517, f=w515) -> (s? t:f=w514:string)
        n408 = flat-sequence {
          tunnel: w514 -> [_]
          frame #0 {
            w525 = 0
            n409 = local write "ScratchPads"(w525) -> ()
            n410 = local write "New Test"(w525) -> ()
          }
        }
        n411 = call "ScratchOrNew.vi"("Template"=w514) -> ("Success"=w522:bool, "Settings Out"=w521:T12)  [unwired: 9 in]
        n412 = case shown="True" w522 {
          tunnel: w521 -> [_ w529]
          tunnel: w511 -> [_ w528]
          tunnel: w520 -> [_ w527]
          frame False {
          }
          frame True {
            n413 = call "Curtin1_Acquire.vi"("MainVI"=w527, "Settings"=w529) -> ("Data?"=w526:bool)  [unwired: 7 in, 2 out]
            n414 = case shown="True" w526 {
              tunnel: w528 -> [_ w531]
              frame False {
                # "No data taken"
                n415 = call "Ask_delete.vi"() -> ()  [unwired: 12 in]
              }
              frame True {
                # "success"
                n416 = Enqueue Element(queue=w531, element="AppendTest") -> ()  [unwired: 2 in, 3 out]
              }
            }
          }
        }
      }
      event "Start": Value Change {
        n417 = event-data() -> ()  [unwired: 1 in, 1 out]
        n418 = call "Startup Wizard.vi"() -> ("analysis?"=w532:string, "Settings"=w533:T12)  [unwired: 10 in]
        n419 = case shown="\"acq\"" w532 {
          tunnel: w535 -> [w539 w543 _]
          tunnel: w534 -> [w538 _ _]
          tunnel: w533 -> [w537 _ _]
          frame "acq" {
            n420 = call "Curtin1_Acquire.vi"("MainVI"=w538, "Settings"=w537) -> ("Data?"=w536:bool)  [unwired: 7 in, 2 out]
            n421 = case shown="True" w536 {
              tunnel: w539 -> [_ w541]
              frame False {
                # "No data taken"
                n422 = call "Ask_delete.vi"() -> ()  [unwired: 12 in]
              }
              frame True {
                n423 = Enqueue Element(queue=w541, element="AppendTest") -> ()  [unwired: 2 in, 3 out]
              }
            }
          }
          frame "analysis" {
            n424 = Enqueue Element(queue=w543, element="Preload") -> ()  [unwired: 2 in, 3 out]
          }
          frame Default {
          }
        }
      }
      event "Help": Value Change {
        n425 = event-data() -> ()  [unwired: 1 in, 1 out]
        n426 = fn#1354() -> (1:w545:bool)  [unwired: 1 out]
        n427 = Not(x=w545) -> (.not. x?=w544:bool)
        n428 = Control Help Window(1:w544) -> ()  [unwired: 1 in]
      }
      event "Preferences": Value Change {
        n429 = event-data() -> ()  [unwired: 1 in, 1 out]
        n430 = call "Curtin_MouseBusy.vi"("VI in"=w547, "element"="Preferences", "queue in"=w548) -> ()  [unwired: 8 in, 1 out]
      }
      event "Settings": Value Change {
        w549 = u16 0 items=["Settings...", "Preferences", "Templates", "Calibrations"] ("Settings")
        n431 = event-data() -> ()  [unwired: 1 in, 1 out]
        n432 = Index Array(array=string[] ["", "Preferences", "Templates", "Calibrations", "LiveView", "MotorControl"], index="Settings") -> (element=w550:string)
        n433 = Enqueue Element(queue=w553, element=w550) -> ()  [unwired: 2 in, 3 out]
        n434 = local write "Settings"(w549) -> ()
      }
      event "zoom": Value Change {
        n435 = event-data() -> ()  [unwired: 1 in, 1 out]
        n436 = Enqueue Element(queue=w555, element="Zoom") -> ()  [unwired: 2 in, 3 out]
      }
      event "email": Value Change {
        n437 = event-data() -> ()  [unwired: 1 in, 1 out]
        n438 = call-poly <vilib>:"Open URL in Default Browser.vi"("URL"="https://sites.google.com/view/oberlinacoustics/contactbug-reports") -> ()  [unwired: 5 in, 2 out]
      }
      event "About": Value Change {
        n439 = event-data() -> ()  [unwired: 1 in, 1 out]
        n440 = call "ObieHelp.vi"() -> ()  [unwired: 12 in]
      }
      event "Interpret": Value Change {
        n441 = event-data() -> ()  [unwired: 1 in, 1 out]
        n442 = property on="Bands" class="Ring (strict)"() -> ("Value"=w559:u16)  [unwired: 2 in, 2 out]
        n443 = local read "FRF"() -> (w557:cluster{"x0":dbl, "df":dbl, dbl[]}[])
        n444 = case shown="Default" w559 {
          tunnel: [w560 w561] -> w558
          tunnel: w557 -> [w560 w563]
          frame 0 {
          }
          frame Default {
            n445 = Array Size(array=w563) -> (size(s)=w564:i32)
            n446 = expression code="x*2/3"(w564) -> (w562:i32)
            n447 = Split 1D Array(array=w563, index=w562) -> (second subarray=w561:cluster{"x0":dbl, "df":dbl, dbl[]}[])  [unwired: 1 out]
          }
        }
        n448 = call "Explainations.vi"("FRF"=w558) -> ()  [unwired: 11 in]
      }
      event "Fun": Value Change {
        n449 = event-data() -> ()  [unwired: 1 in, 1 out]
        n450 = Enqueue Element(queue=w565, element="Fun") -> ()  [unwired: 2 in, 3 out]
      }
      event "microphone": Value Change {
        (unwired) "Preferences" ("element")
        n451 = event-data() -> ()  [unwired: 1 in, 1 out]
        n452 = call "Curtin_MouseBusy.vi"("VI in"=w571, "element"="LiveView", "queue in"=w570) -> ()  [unwired: 8 in, 1 out]
        n453 = property on="Device" class="Ring (strict)"("Strings []"=string[] ["Initializing..."] ("Strings [4]"), "Value"=0) -> ()  [unwired: 2 in, 2 out]
      }
      event "FRF": Shortcut Menu Activation? {
        n454 = event-data() -> ("MenuRef"=w575:refnum<k9>)  [unwired: 1 in]
        n455 = property on="Bands" class="Ring (strict)"() -> ("Value"=w572:u16)  [unwired: 2 in, 2 out]
        n456 = property on="View Type" class="Ring (strict)"() -> ("Value"=w573:u16)  [unwired: 2 in, 2 out]
        n457 = call "GenerateMenuItems.vi"("Bands"=w572, "View Type"=w573, "Menu in"=w575) -> ("error out"=w574:errorcluster)  [unwired: 8 in]
        n458 = event-data() -> ()  [unwired: 2 in, 1 out]
      }
      event "FRF": Shortcut Menu Selection (User) {
        n459 = event-data() -> ("CtlRef"=w576:refnum<vi>, "ItemTag"=w578:string)  [unwired: 1 in]
        n460 = case shown="\"toggleCentroids\"" w578 {
          tunnel: w577 -> [_ w579 _ _ _ w589 w592 _ _ w595 w597 w599 _]
          tunnel: w576 -> [_ _ w585 w586 _ _ _ _ _ _ _ _ _]
          frame Default {
          }
          frame "toggleCentroids" {
            n461 = global read "Mic_Global.vi" "View"() -> (w583:T9)
            n462 = Unbundle By Name(w583) -> ("Centroids?"=w584:bool)
            n463 = Enqueue Element(queue=w579, element="Update") -> ()  [unwired: 2 in, 3 out]
            n464 = Not(x=w584) -> (.not. x?=w582:bool)
            n465 = Bundle By Name(cluster=w583, "Centroids?"=w582) -> (w581:T9)
            n466 = global write "Mic_Global.vi" "View"(w581) -> ()
          }
          frame "savePlot" {
            n467 = call "ExportPlots.vi"("WaveformGraph in"=w585) -> ()  [unwired: 11 in]
          }
          frame "copyImage" {
            n468 = call "GrabPlotImage.vi"("WaveformGraph in"=w586) -> ()  [unwired: 11 in]
          }
          frame "autoScale" {
            n469 = property on="dB Range" class="DigNum (strict)"() -> ("Value"=w588:dbl)  [unwired: 2 in, 2 out]
            n470 = call "AutoscaleYaxis.vi"("Has Coherence in plot?"=FALSE, "dB Range"=w588) -> ()  [unwired: 10 in]
          }
          frame "Folder" {
            n471 = Enqueue Element(queue=w589, element="Folder") -> ()  [unwired: 2 in, 3 out]
          }
          frame "saveGroup" {
            n472 = Enqueue Element(queue=w592, element="AppendAve") -> ()  [unwired: 2 in, 3 out]
          }
          frame "FontAdjust" {
            n473 = control-ref of="FRF"() -> (w593:refnum<vi>)
            n474 = call "Ask_Font.vi"("WaveformGraph in"=w593) -> ()  [unwired: 11 in]
          }
          frame "MATLAB" {
            n475 = control-ref of="FRF"() -> (w594:refnum<vi>)
            n476 = call "MATLAB.vi"("Graph"=w594) -> ()  [unwired: 10 in, 1 out]
          }
          frame "WOOD" {
            n477 = Enqueue Element(queue=w595, element="woodhouse") -> ()  [unwired: 2 in, 3 out]
          }
          frame "SAM" {
            n478 = Enqueue Element(queue=w597, element="SamZ") -> ()  [unwired: 2 in, 3 out]
          }
          frame "PLAY" {
            n479 = Enqueue Element(queue=w599, element="PlayIt") -> ()  [unwired: 2 in, 3 out]
          }
          frame "Trends" {
            n480 = control-ref of="FRF"() -> (w603:refnum<vi>)
            n481 = property on="Bands" class="Ring (strict)"() -> ("Value"=w602:u16)  [unwired: 2 in, 2 out]
            n482 = Not Equal To 0?(x=w602) -> (x != 0?=w601:bool)
            n483 = call "PlotBandsAgainstRun.vi"("Bands?"=w601, "Graph"=w603) -> ()  [unwired: 10 in]
          }
        }
      }
    }
  }
  n484 = disable-structure shown="Default" {
    disable-tunnel: [_ TRUE] -> w9
    frame condition #0 (active) {
    }
    frame condition #1 {
    }
  }
  n485 = property on="Position" class="Str"("Text.FontBold"=w9) -> ()  [unwired: 2 in, 2 out]
  n486 = disable-structure shown="RUN_TIME_ENGINE==True" {
    disable-tunnel: w8 -> [_ _]
    frame condition #0 (active) {
    }
    frame condition #1 {
      # "Stop everytng from running"
      n487 = control-ref of="This VI"() -> (w606:refnum<vi>)
      n488 = property class="VI"("FP.State"=T15."Closed" ("Front Panel Window:State")) -> (error out=w605:errorcluster)  [unwired: 2 in, 1 out]
      n489 = invoke class="VI" method="Abort VI"(reference=w606, error in=w605) -> ()  [unwired: 1 in, 3 out]
    }
  }
